vi "阵型选择.vi"(0 "选择阵列":enum16{"圆形阵列 32阵元"}(ring)) -> (14 "阵列形状：":cluster{dbl[], dbl[]}(graph))   [LabVIEW 2018]
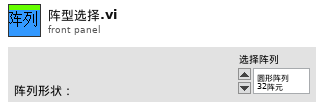
[diagram p1: front panel]
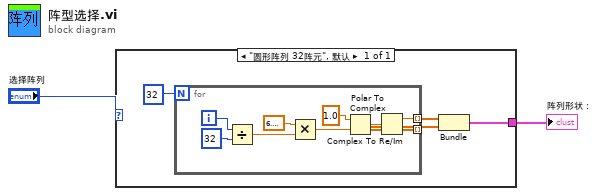
[diagram p0: block diagram]
diagram:
  n1 = case shown="\"圆形阵列 32阵元\", 默认" "选择阵列" {
    tunnel: [w4] -> w1
    frame "圆形阵列 32阵元", Default {
      n2 = for {
        N: 32 -> [_]
        tunnel: [w13] -> w6 mode=indexing
        tunnel: [w12] -> w5 mode=indexing
        i -> [w11]
        n3 = Divide(x=w11, y=32) -> (x/y=w9:dbl)
        n4 = Multiply(x=6.283185307179586, y=w9) -> (x*y=w8:dbl)
        n5 = Polar To Complex(1:w8, 2:1.0 ("r")) -> (0:w14:cdb)
        n6 = Complex To Re/Im(x + iy=w14) -> (x=w13:dbl, y=w12:dbl)
      }
      n7 = Bundle(w6, w5) -> (w4:cluster{dbl[], dbl[]})  [unwired: 1 in]
    }
  }
  "阵列形状：" <- w1
